vi "cluster_to_settings_ini_file.vi"(8 "error in (no error)":errorcluster, 11 "containerIn":variant) -> (0 "error out":errorcluster)   [LabVIEW 2015, in "ini_work_Library.lvlib"]
doc: "Write any cluster to data/settings.ini file\n\nCreated by Artem Shevelev\nshevelev.pro\nartem@shevelev.pro\nLabVIEW Portal: https://labviewportal.org/memberlist.php?mode=viewprofile&u=2340"
uses:
  ini_work_Library.lvlib
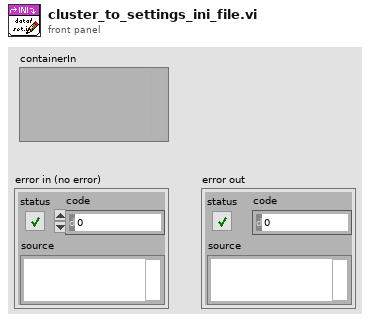
[diagram p1: front panel]
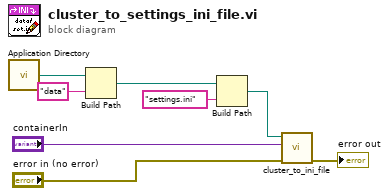
[diagram p0: block diagram]
diagram:
  n1 = call <vilib>:"Application Directory.vi"() -> ("Application Directory"=w4:path)
  n2 = Build Path(base path=w4, name or relative path="data") -> (appended path=w2:path)
  n3 = Build Path(base path=w2, name or relative path="settings.ini") -> (appended path=w3:path)
  n4 = call "cluster_to_ini_file.vi"("error in (no error)"="error in (no error)", "data"="containerIn", "iniFilePath"=w3) -> ("error out"=→"error out":errorcluster)  [unwired: 8 in]
